vi "SQL Select.vi"(8 "error in (no error)":errorcluster, 10 "Select Statement":string, 11 "Database Name":string) -> (0 "error out":errorcluster, 1 "Select Result":string[][](array[string]), 2 "Select Fields":string[](array[string]), 3 "return code":i32)   [LabVIEW 2011]
doc: "Provides a simple select API to SQLite. The return code is determined by the SQLite Engine, and could be used to genertate a custom LabVIEW error. For more information on the SQLite query formats and erorrs please search to the SQLite documentation."
uses:
  SQLite Source/CVI RT/sqlitewrapper.dll
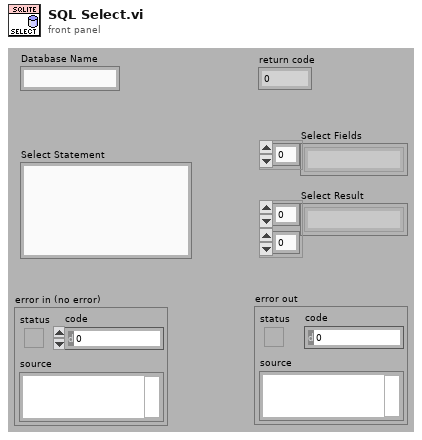
[diagram p1: front panel]
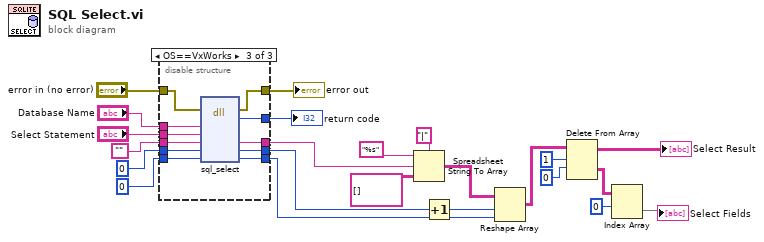
[diagram p0: block diagram]
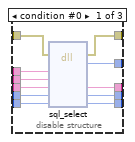
[diagram p2: hidden frame]
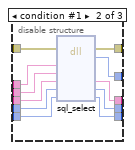
[diagram p3: hidden frame]
diagram:
  n1 = disable-structure shown="OS==VxWorks" {
    disable-tunnel: 0 ("rows") -> [w34 w40 w56]
    disable-tunnel: 0 ("cols") -> [w33 w39 w55]
    disable-tunnel: "Database Name" -> [w32 w43 w54]
    disable-tunnel: "Select Statement" -> [w31 w42 w53]
    disable-tunnel: [w30 w35 w52] -> w19
    disable-tunnel: [w29 w37 w51] -> w1
    disable-tunnel: [w28 w38 w50] -> w11
    disable-tunnel: [w27 w36 w49] -> w10
    disable-tunnel: "" -> [w26 w41 w48]
    disable-tunnel: "error in (no error)" -> [w25 w45 w47]
    disable-tunnel: [w24 w44 w46] -> w16
    frame condition #0 {
      n2 = dll-call lib="C:/Git/B2G/lv_sqlite_103/SQLite Source/CVI RT/sqlitewrapper.*" fn="sql_select"(error in=w25, "dbName"=w32, "statement"=w31, "result_string"=w26, "rows"=w34, "cols"=w33) -> (error out=w24:errorcluster, "return type"=w30:i32, "result_string"=w27:string, "rows"=w29:i32, "cols"=w28:i32)  [unwired: 4 in, 1 out]
    }
    frame condition #1 {
      n3 = dll-call lib="C:/Git/B2G/lv_sqlite_103/SQLite Source/CVI RT/sqlitewrapper.dll" fn="sql_select"(error in=w45, "dbName"=w43, "statement"=w42, "result_string"=w41, "rows"=w40, "cols"=w39) -> (error out=w44:errorcluster, "return type"=w35:i32, "result_string"=w36:string, "rows"=w37:i32, "cols"=w38:i32)  [unwired: 4 in, 1 out]
    }
    frame condition #2 (active) {
      n4 = dll-call lib="C:/Git/B2G/lv_sqlite_103/SQLite Source/CVI RT/sqlitewrapper.*" fn="sql_select"(error in=w47, "dbName"=w54, "statement"=w53, "result_string"=w48, "rows"=w56, "cols"=w55) -> (error out=w46:errorcluster, "return type"=w52:i32, "result_string"=w49:string, "rows"=w51:i32, "cols"=w50:i32)  [unwired: 4 in, 1 out]
    }
  }
  "return code" <- w19
  "error out" <- w16
  n5 = Spreadsheet String To Array(delimiter (Tab)="|", format string="%s", spreadsheet string=w10, array type (2D Dbl)=string[][] []) -> (array=w13:string[][])
  n6 = Increment(x=w1) -> (x+1=w2:i32)
  n7 = Reshape Array(w13, w2, w11) -> (w9:string[][])
  n8 = Delete From Array(array=w9, length=1, index (row)=0) -> (deleted portion=w5:string[][], array with subset deleted=→"Select Result":string[][])  [unwired: 1 in]
  n9 = Index Array(array=w5, index (row)=0) -> (element=→"Select Fields":string[])  [unwired: 1 in]
